vi "DeviceUI.vi"() -> ()   [LabVIEW 2014, in "Device.lvclass"]
doc: "UI that will be called when the node is selected."
uses:
  Device.lvclass
  <vilib>/NI/Configuration Framework/Node/NodeRef.ctl
  <vilib>/NI/Configuration Framework/Node/NISE_CEF_Node.lvclass
  <vilib>/NI/AMC/Message Queue.ctl
  <vilib>/NI/AMC/Message.ctl
  <vilib>/NI/Tools/Keyed Array/KeyedArray.ctl
  <vilib>/NI/Configuration Framework/Node/UserEventRef.ctl
  <vilib>/NI/Configuration Framework/Controls/EventCluster.ctl
  Bus/Bus.lvclass
  <vilib>/NI/Configuration Framework/Node/NISE_CEF_Node.lvclass/NISE_CEF_Node.ctl
  Device.lvclass/Device.ctl
  Device Configuration/Device Configuration.lvclass/Device Configuration.ctl
  RIO Target/RIO Target.lvclass
  RIO Target Configuration/RIO Target Configuration.lvclass
  <vilib>/NI/AMC/Create Single Message.vi
  <vilib>/NI/AMC/Update Message Routing Info.vi
  <vilib>/NI/Configuration Framework/serializable configuration/read metadata property.vi
  <vilib>/NI/AMC/Send Message.vi
  <vilib>/NI/Configuration Framework/serializable configuration/set metadata property.vi
  <vilib>/NI/AMC/AMC.lvlib
  <vilib>/NI/Configuration Framework/serializable configuration/NISE_CEF_serializable configuration.lvclass
  Device Configuration/Device Configuration.lvclass
  <vilib>/NI/Tools/Keyed Array/Tools_KeyedArray.lvlib
  <vilib>/NI/Configuration Framework/NISE_CEF_TreeControl.lvlib
panel:
  in  "Device Icon Name":string
  in  "Number of Channels":u32
  in  "Chip Select":string(combo)
  in  "Description":string
  in  "Alias":string
  in  "user event":T1
  in  "main queue":T2
  in  "node ref":T3
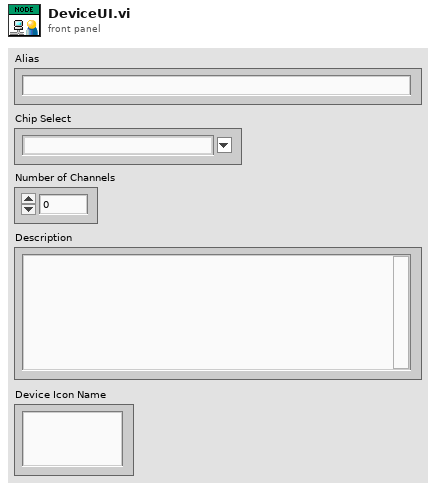
[diagram p1: front panel]
types:
  T1 = typedef "NISE_CEF_Node.lvclass/UserEventRef.ctl" = refnum<user-event>
  T2 = typedef "AMC.lvlib/Message Queue.ctl" = refnum<queue>
  T3 = typedef "NISE_CEF_Node.lvclass/NodeRef.ctl" = refnum<data-value>
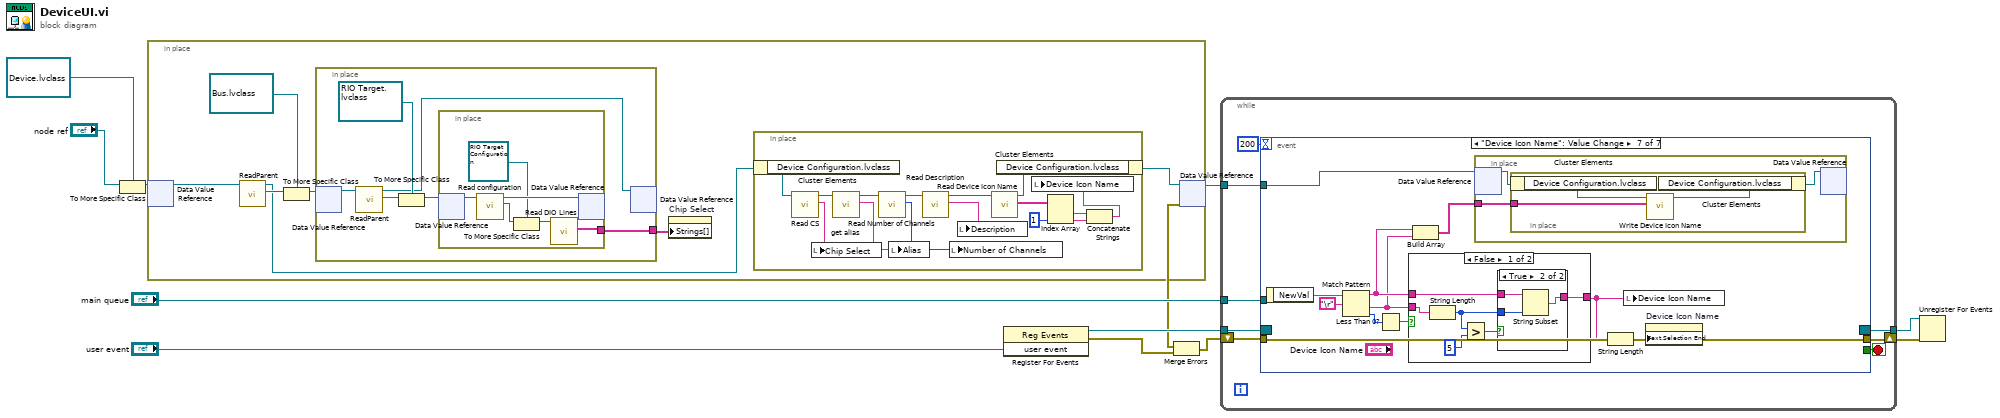
[diagram p0: block diagram]
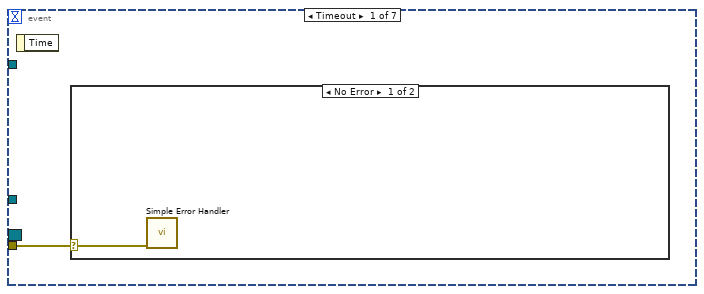
[diagram p2: hidden frame]
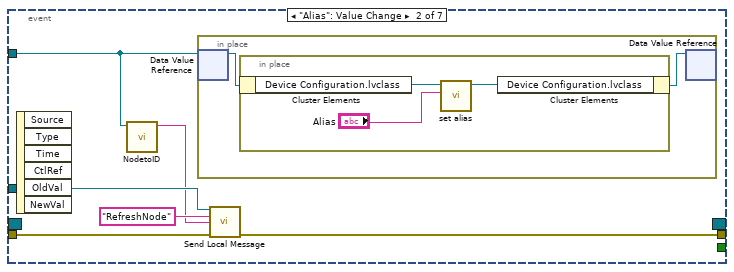
[diagram p4: hidden frame]
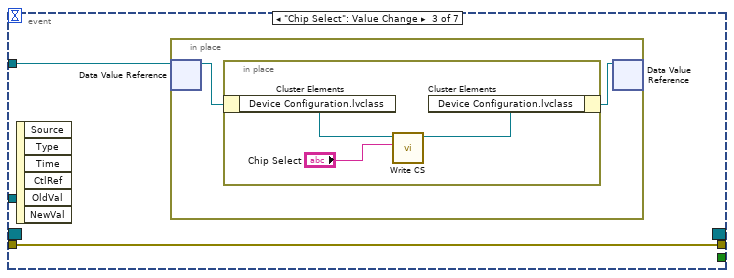
[diagram p5: hidden frame]
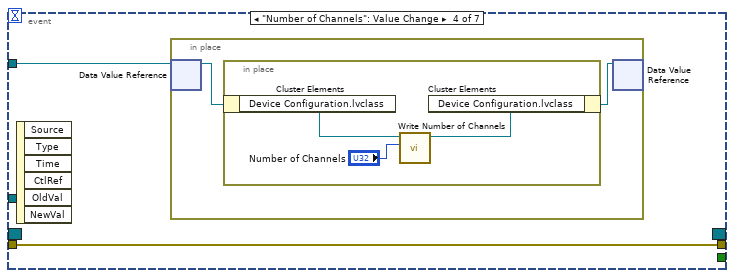
[diagram p6: hidden frame]
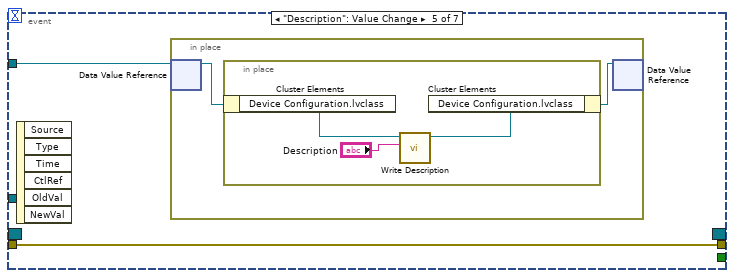
[diagram p7: hidden frame]
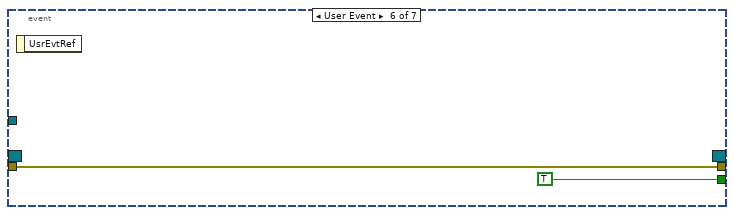
[diagram p8: hidden frame]
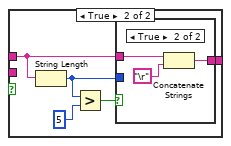
[diagram p10: hidden frame]
diagram:
  n1 = To More Specific Class(target class=refnum<data-value> refnum ("data value reference"), reference="node ref") -> (specific class reference=w1:refnum<data-value>)  [unwired: 1 in, 1 out]
  n2 = in-place {
    n3 = in-place-dvr #1(w1) -> (w16:refnum<class "Device.lvclass">)  [unwired: 1 out]
    n4 = call <vilib>:"ReadParent.vi"("node in"=w16) -> ("parent"=w19:T3, "node out"=w14:refnum<class "Device.lvclass">)  [unwired: 8 in, 1 out]
    n5 = To More Specific Class(target class=refnum<data-value> refnum ("data value reference"), reference=w19) -> (specific class reference=w17:refnum<data-value>)  [unwired: 1 in, 1 out]
    n6 = in-place {
      in-place-border: [w37] -> w13
      n7 = in-place-dvr #2(w17) -> (w38:refnum<class "Bus.lvclass">)  [unwired: 1 out]
      n8 = call <vilib>:"ReadParent.vi"("node in"=w38) -> ("parent"=w40:T3, "node out"=w36:refnum<class "Bus.lvclass">)  [unwired: 8 in, 1 out]
      n9 = To More Specific Class(target class=refnum<data-value> refnum ("data value reference"), reference=w40) -> (specific class reference=w35:refnum<data-value>)  [unwired: 1 in, 1 out]
      n10 = in-place {
        in-place-border: [w41] -> w37
        n11 = in-place-dvr #3(w35) -> (w46:refnum<class "RIO Target.lvclass">)  [unwired: 1 out]
        n12 = call-dynamic "Read configuration.vi"("RIO Target in"=w46) -> ("configuration"=w44:refnum<class "NISE_CEF_serializable configuration.lvclass">, "RIO Target out"=w45:refnum<class "RIO Target.lvclass">)  [unwired: 8 in, 1 out]
        n13 = To More Specific Class(target class=refnum<class "RIO Target Configuration.lvclass"> refnum ("RIO Target Configuration in"), reference=w44) -> (specific class reference=w42:refnum<class "RIO Target Configuration.lvclass">)  [unwired: 1 in, 1 out]
        n14 = call "Read DIO Lines.vi"("RIO Target Configuration in"=w42) -> ("DIO Lines"=w41:string[])  [unwired: 8 in, 2 out]
        n15 = in-place-dvr #3(w45) -> ()  [unwired: 2 out]
      }
      n16 = in-place-dvr #2(w36) -> ()  [unwired: 2 out]
    }
    n17 = property on="Chip Select" class="CmbBox"("Strings[]"=w13) -> ()  [unwired: 2 in, 2 out]
    n18 = in-place {
      n19 = in-place-cluster #4(w14) -> ("Device Configuration.lvclass"=w34:refnum<class "Device Configuration.lvclass">)
      n20 = call "Read CS.vi"("Device Configuration in"=w34) -> ("CS"=w32:string, "Device Configuration out"=w33:refnum<class "Device Configuration.lvclass">)  [unwired: 8 in, 1 out]
      n21 = local write "Chip Select"(w32) -> ()
      n22 = call <vilib>:"get alias.vi"("configuration in"=w33) -> ("alias"=w31:string, "configuration out"=w30:refnum<class "Device Configuration.lvclass">)  [unwired: 8 in, 1 out]
      n23 = call "Read Number of Channels.vi"("Device Configuration in"=w30) -> ("Number of Channels"=w29:u32, "Device Configuration out"=w28:refnum<class "Device Configuration.lvclass">)  [unwired: 8 in, 1 out]
      n24 = local write "Alias"(w31) -> ()
      n25 = call "Read Description.vi"("Device Configuration in"=w28) -> ("Description"=w27:string, "Device Configuration out"=w26:refnum<class "Device Configuration.lvclass">)  [unwired: 8 in, 1 out]
      n26 = local write "Number of Channels"(w29) -> ()
      n27 = local write "Description"(w27) -> ()
      n28 = call "Read Device Icon Name.vi"("Device Configuration in"=w26) -> ("Device Icon Name"=w24:string[], "Device Configuration out"=w25:refnum<class "Device Configuration.lvclass">)  [unwired: 8 in, 1 out]
      n29 = in-place-cluster #4("Device Configuration.lvclass"=w25) -> (w15:refnum<class "Device.lvclass">)
      n30 = Index Array(array=w24, index #2=1 ("index")) -> (element #1=w22:string, element #2=w21:string)  [unwired: 1 in]
      n31 = Concatenate Strings(w22, w21) -> (w20:string)
      n32 = local write "Device Icon Name"(w20) -> ()
    }
    n33 = in-place-dvr #1(w15) -> (w12:refnum<data-value>, w6:errorcluster)
  }
  n34 = register-events("user event") -> (reference out=w9:refnum<event-registration>, error out=w5:errorcluster)  [unwired: 2 in]
  n35 = Merge Errors(w6, w5) -> (w4:errorcluster)
  n36 = while {
    tunnel: w12 -> [w54]
    tunnel: "main queue" -> [w53]
    tunnel: w9 -> [w51]
    tunnel: [w50] -> w8
    shift-right: [w48] -> w7
    shift-left: w4 -> [w47]
    stop <- w49 stop-if-true
    n37 = event shown="[6] \"Device Icon Name\": Value Change" {
      selector: w51 -> [_ _ _ _ _ _ _]
      dyn-events: [_ _ _ _ _ _ _] -> w50
      timeout: 200 -> [_ _ _ _ _ _ _]
      tunnel: w54 -> [_ w57 w68 w75 w82 _ w95]
      tunnel: w53 -> [_ w61 _ _ _ _ _]
      tunnel: [_ _ _ _ _ TRUE _] -> w49
      tunnel: [_ w59 w69 w76 w83 w89 w101] -> w48
      tunnel: w47 -> [w55 w58 w69 w76 w83 w89 w101]
      event Timeout {
        n38 = event-data() -> ()  [unwired: 1 in, 1 out]
        n39 = case shown="No Error" w55 {
          selector: w55 -> [w56 _]
          frame No Error {
            n40 = call <vilib>:"Simple Error Handler.vi"("error in (no error)"=w56) -> ()  [unwired: 4 in, 5 out]
          }
          frame Error {
          }
        }
      }
      event "Alias": Value Change {
        n41 = event-data() -> ()  [unwired: 1 in, 6 out]
        n42 = call <vilib>:"NodetoID.vi"("node ref"=w57) -> ("ID"=w60:string)  [unwired: 9 in, 1 out]
        n43 = in-place {
          n44 = in-place-dvr #5(w57) -> (w64:refnum<class "Device.lvclass">)  [unwired: 1 out]
          n45 = in-place {
            n46 = in-place-cluster #6(w64) -> ("Device Configuration.lvclass"=w67:refnum<class "Device Configuration.lvclass">)
            n47 = call <vilib>:"set alias.vi"("alias"="Alias", "configuration in"=w67) -> ("configuration out"=w66:refnum<class "Device Configuration.lvclass">)  [unwired: 8 in, 1 out]
            n48 = in-place-cluster #6("Device Configuration.lvclass"=w66) -> (w63:refnum<class "Device.lvclass">)
          }
          n49 = in-place-dvr #5(w63) -> ()  [unwired: 2 out]
        }
        n50 = call <vilib>:"Send Local Message.vi"("message queue in"=w61, "message name"="RefreshNode" ("Message Name"), "message value"=w60, "error in"=w58) -> ("error out"=w59:errorcluster)  [unwired: 9 in, 2 out]
      }
      event "Chip Select": Value Change {
        n51 = event-data() -> ()  [unwired: 1 in, 6 out]
        n52 = in-place {
          n53 = in-place-dvr #7(w68) -> (w71:refnum<class "Device.lvclass">)  [unwired: 1 out]
          n54 = in-place {
            n55 = in-place-cluster #8(w71) -> ("Device Configuration.lvclass"=w74:refnum<class "Device Configuration.lvclass">)
            n56 = call "Write CS.vi"("CS"="Chip Select", "Device Configuration in"=w74) -> ("Device Configuration out"=w73:refnum<class "Device Configuration.lvclass">)  [unwired: 8 in, 1 out]
            n57 = in-place-cluster #8("Device Configuration.lvclass"=w73) -> (w70:refnum<class "Device.lvclass">)
          }
          n58 = in-place-dvr #7(w70) -> ()  [unwired: 2 out]
        }
      }
      event "Number of Channels": Value Change {
        n59 = event-data() -> ()  [unwired: 1 in, 6 out]
        n60 = in-place {
          n61 = in-place-dvr #9(w75) -> (w78:refnum<class "Device.lvclass">)  [unwired: 1 out]
          n62 = in-place {
            n63 = in-place-cluster #10(w78) -> ("Device Configuration.lvclass"=w81:refnum<class "Device Configuration.lvclass">)
            n64 = call "Write Number of Channels.vi"("Number of Channels"="Number of Channels", "Device Configuration in"=w81) -> ("Device Configuration out"=w80:refnum<class "Device Configuration.lvclass">)  [unwired: 8 in, 1 out]
            n65 = in-place-cluster #10("Device Configuration.lvclass"=w80) -> (w77:refnum<class "Device.lvclass">)
          }
          n66 = in-place-dvr #9(w77) -> ()  [unwired: 2 out]
        }
      }
      event "Description": Value Change {
        n67 = event-data() -> ()  [unwired: 1 in, 6 out]
        n68 = in-place {
          n69 = in-place-dvr #11(w82) -> (w85:refnum<class "Device.lvclass">)  [unwired: 1 out]
          n70 = in-place {
            n71 = in-place-cluster #12(w85) -> ("Device Configuration.lvclass"=w88:refnum<class "Device Configuration.lvclass">)
            n72 = call "Write Description.vi"("Description"="Description", "Device Configuration in"=w88) -> ("Device Configuration out"=w87:refnum<class "Device Configuration.lvclass">)  [unwired: 8 in, 1 out]
            n73 = in-place-cluster #12("Device Configuration.lvclass"=w87) -> (w84:refnum<class "Device.lvclass">)
          }
          n74 = in-place-dvr #11(w84) -> ()  [unwired: 2 out]
        }
      }
      event User Event {
        n75 = event-data() -> ()  [unwired: 1 in, 1 out]
      }
      event "Device Icon Name": Value Change {
        n76 = event-data() -> ("NewVal"=w100:string)  [unwired: 1 in]
        n77 = Match Pattern(string=w100, regular expression="\r") -> (before substring=w93:string, after substring=w92:string, offset past match=w98:i32)  [unwired: 1 in, 1 out]
        n78 = Less Than 0?(x=w98) -> (x < 0?=w97:bool)
        n79 = case shown="False" w97 {
          tunnel: w93 -> [w111 w120]
          tunnel: w92 -> [w108 _]
          tunnel: [w109 w118] -> w94
          frame False {
            n80 = String Length(string=w108) -> (length=w110:i32)
            n81 = Greater?(x=w110, y=5) -> (0:w112:bool)
            n82 = case shown="True" w112 {
              tunnel: w111 -> [w114 w117]
              tunnel: w110 -> [_ w115]
              tunnel: [w114 w116] -> w109
              frame False {
              }
              frame True {
                n83 = String Subset(string=w117, length (rest)=w115) -> (substring=w116:string)  [unwired: 1 in]
              }
            }
          }
          frame True {
            n84 = String Length(string=w120) -> (length=w119:i32)
            n85 = Greater?(x=w119, y=5) -> (0:w121:bool)
            n86 = case shown="True" w121 {
              tunnel: w120 -> [w123 w126]
              tunnel: w119 -> [_ _]
              tunnel: [w123 w124] -> w118
              frame False {
              }
              frame True {
                n87 = Concatenate Strings(w126, "\r") -> (w124:string)
              }
            }
          }
        }
        n88 = Build Array(w93, w92) -> (w91:string[])
        n89 = in-place {
          in-place-border: w91 -> [w102]
          n90 = in-place-dvr #13(w95) -> (w104:refnum<class "Device.lvclass">)  [unwired: 1 out]
          n91 = in-place {
            in-place-border: w102 -> [w105]
            n92 = in-place-cluster #14(w104) -> ("Device Configuration.lvclass"=w107:refnum<class "Device Configuration.lvclass">)
            n93 = call "Write Device Icon Name.vi"("Device Icon Name"=w105, "Device Configuration in"=w107) -> ("Device Configuration out"=w106:refnum<class "Device Configuration.lvclass">)  [unwired: 8 in, 1 out]
            n94 = in-place-cluster #14("Device Configuration.lvclass"=w106) -> (w103:refnum<class "Device.lvclass">)
          }
          n95 = in-place-dvr #13(w103) -> ()  [unwired: 2 out]
        }
        n96 = String Length(string=w94) -> (length=w96:i32)
        n97 = local write "Device Icon Name"(w94) -> ()
        n98 = property on="Device Icon Name" class="Str"("Text.Selection End"=w96) -> ()  [unwired: 2 in, 2 out]
      }
    }
  }
  n99 = Unregister For Events(event registration refnum=w8, error in=w7) -> ()  [unwired: 1 out]
